vi "Excel_Picture.vi"(7 "references":T1, 8 "error in":errorcluster, 9 "End(-1,-1)":cluster{"row":i32, "column":i32}, 10 "start(-1,-1)":cluster{"row":i32, "column":i32}, 11 "Picture Path":path) -> (0 "error out":errorcluster, 3 "Workbook":refnum<k7>)   [LabVIEW 2011]
doc: "自己改的，向Excel表格中添加图片"
uses:
  <vilib>/addons/_office/NI_ReportGenerationToolkit.lvlib
panel:
  in  "name":string
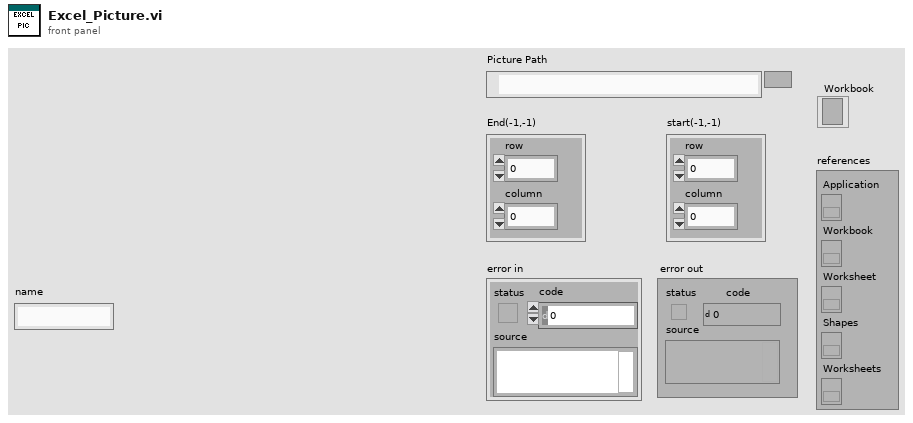
[diagram p1: front panel]
types:
  T1 = cluster{"Application":refnum<k7>, "Workbook":refnum<k7>, "Worksheet":refnum<k7>, "Shapes":refnum<k7>, "Worksheets":refnum<k7>}
  T2 = typedef "imagedata.ctl" = cluster{"image type":i32, "image depth":i32, "image":u8[], "mask":u8[], "colors":u32[], "Rectangle":cluster{"left":i16, "top":i16, "right":i16, "bottom":i16}}
  T3 = cluster{"left":i16, "top":i16, "right":i16, "bottom":i16}
  T4 = cluster{"left":dbl, "top":dbl, "right":dbl, "bottom":dbl}
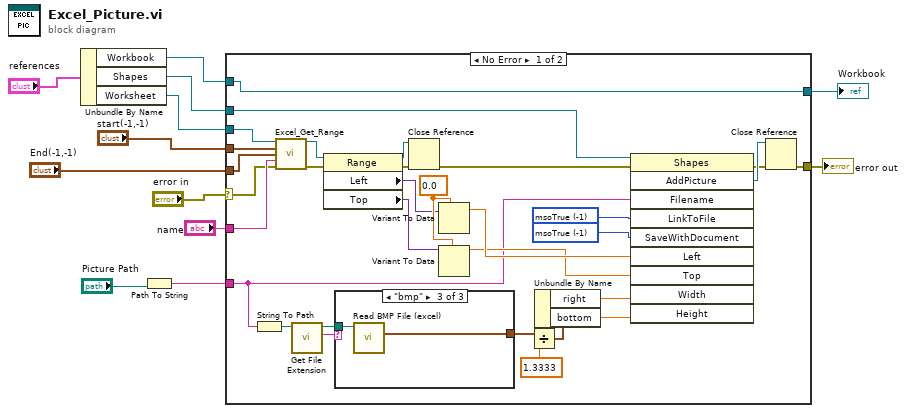
[diagram p0: block diagram]
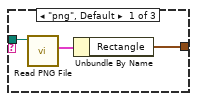
[diagram p2: hidden frame]
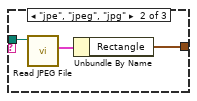
[diagram p3: hidden frame]
diagram:
  n1 = Unbundle By Name("references") -> ("Workbook"=w2:refnum<k7>, "Shapes"=w8:refnum<k7>, "Worksheet"=w7:refnum<k7>)
  n2 = Path To String(path="Picture Path") -> (string=w10:string)
  n3 = case shown="No Error" "error in" {
    selector: "error in" -> [w21 w53]
    tunnel: [w41 w53] -> w12
    tunnel: w10 -> [w32 _]
    tunnel: w7 -> [w23 _]
    tunnel: "name" -> [w22 _]
    tunnel: w8 -> [w19 _]
    tunnel: "start(-1,-1)" -> [w15 _]
    tunnel: "End(-1,-1)" -> [w14 _]
    tunnel: w2 -> [w13 w52]
    tunnel: [w13 w52] -> w1
    frame No Error {
      w37 = sgl 0.0 ("Left")
      w42 = -1 items=["msoTrue"=-1, "msoFalse"=0, "msoCTrue"=1, "msoTriStateToggle"=-3, "msoTriStateMixed"=-2] ("LinkToFile")
      w43 = -1 items=["msoTrue"=-1, "msoFalse"=0, "msoCTrue"=1, "msoTriStateToggle"=-3, "msoTriStateMixed"=-2] ("SaveWithDocument")
      n4 = String To Path(string=w32) -> (path=w18:path)
      n5 = call <vilib>:"Excel_Get_Range.vi"("Excel._Worksheet"=w23, "start"=w15, "end"=w14, "name"=w22, "error in (no error)"=w21) -> ("Range"=w20:refnum<k7>, "error out"=w24:errorcluster)  [unwired: 9 out]
      n6 = call <vilib>:"Get File Extension.vi"("file"=w18) -> ("lowercase file extension"=w16:string, "dup file"=w17:path)  [unwired: 1 in, 8 out]
      n7 = property class="Range"(reference=w20, error in=w24) -> (reference out=w38:refnum<k7>, error out=w39:errorcluster, "Left"=w36:variant, "Top"=w35:variant)
      n8 = case shown="\"bmp\"" w16 {
        tunnel: w17 -> [w46 w49 w51]
        tunnel: [w44 w47 w50] -> w31
        frame "png", Default {
          n9 = call <vilib>:"Read PNG File.vi"("path to PNG file"=w46) -> ("image data"=w45:T2)  [unwired: 1 in, 9 out]
          n10 = Unbundle By Name(w45) -> ("Rectangle"=w44:T3)
        }
        frame "jpe", "jpeg", "jpg" {
          n11 = call <vilib>:"Read JPEG File.vi"("path to JPEG file"=w49) -> ("image data"=w48:T2)  [unwired: 1 in, 9 out]
          n12 = Unbundle By Name(w48) -> ("Rectangle"=w47:T3)
        }
        frame "bmp" {
          n13 = call <vilib>:"Read BMP File (excel).vi"("path to BMP file"=w51) -> ("rect"=w50:T3)  [unwired: 1 in, 9 out]
        }
      }
      n14 = Close Reference(reference=w38, error in (no error)=w39) -> (error out=w26:errorcluster)
      n15 = Variant To Data(type=w37, Variant=w36) -> (data=w34:sgl)  [unwired: 1 in, 1 out]
      n16 = Variant To Data(type=w37, Variant=w35) -> (data=w33:sgl)  [unwired: 1 in, 1 out]
      n17 = Divide(x=w31, y=1.3333) -> (x/y=w29:T4)
      n18 = Unbundle By Name(w29) -> ("right"=w27:dbl, "bottom"=w28:dbl)
      n19 = invoke class="Shapes" method="AddPicture"(reference=w19, error in=w26, "Filename"=w32, "LinkToFile"=w42, "SaveWithDocument"=w43, "Left"=w34, "Top"=w33, "Width"=w27, "Height"=w28) -> (error out=w25:errorcluster, "AddPicture"=w40:refnum<k7>)  [unwired: 1 in, 8 out]
      n20 = Close Reference(reference=w40, error in (no error)=w25) -> (error out=w41:errorcluster)
    }
    frame Error {
    }
  }
  "error out" <- w12
  "Workbook" <- w1
